vi "PSConverter.vi"(1 "Current States 2":string[][](table), 2 "PROC":string[](array[string]), 3 "STATES":string[][](array[string]), 4 "Input claster":cluster{u32, u8}[](array[cluster])) -> (0 "Current States":string[][](table))   [LabVIEW 2009]
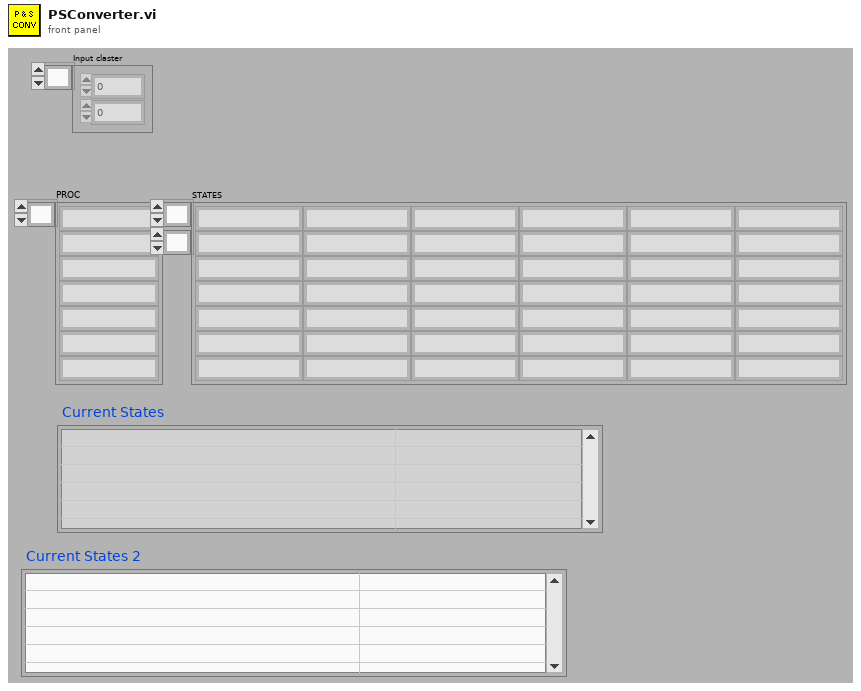
[diagram p1: front panel]
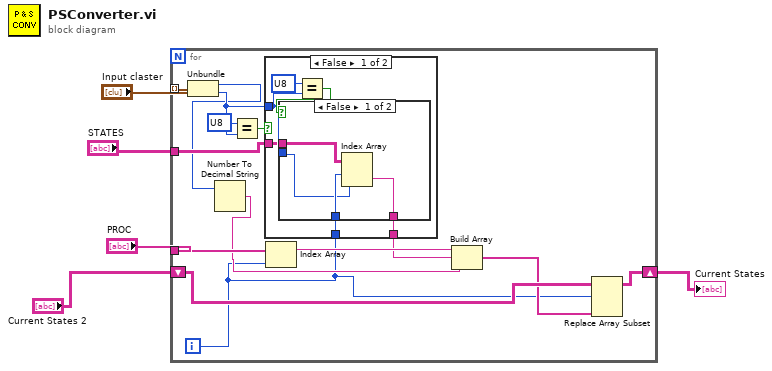
[diagram p0: block diagram]
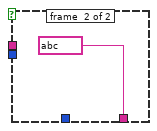
[diagram p2: hidden frame]
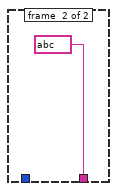
[diagram p3: hidden frame]
diagram:
  n1 = for {
    tunnel: "Input claster" -> [w19] mode=indexing
    tunnel: "PROC" -> [w13]
    tunnel: "STATES" -> [w12]
    shift-right: [w8] -> w5
    shift-left: "Current States 2" -> [w9]
    i -> [w6]
    n2 = Unbundle(w19) -> (w11:u32, w15:u8)
    n3 = Number To Decimal String(number=w11) -> (decimal integer string=w10:string)  [unwired: 1 in]
    n4 = Equal?(x=u8 ?, y=w15) -> (x = y?=w16:bool)
    n5 = case shown="False" w16 {
      tunnel: w15 -> [w21 _]
      tunnel: [w23 string ?] -> w14
      tunnel: w6 -> [w22 _]
      tunnel: w12 -> [w20 _]
      frame #0 {
        n6 = Equal?(x=u8 ?, y=w21) -> (x = y?=w24:bool)
        n7 = case shown="False" w24 {
          tunnel: [w27 string ?] -> w23
          tunnel: w22 -> [w29 _]
          tunnel: w21 -> [w28 _]
          tunnel: w20 -> [w26 _]
          frame #0 {
            n8 = Index Array(array=w26, index (row)=w29, index (col)=w28) -> (element=w27:string)
          }
          frame #1 {
          }
        }
      }
      frame #1 {
      }
    }
    n9 = Index Array(array=w13, index=w6) -> (element=w18:string)
    n10 = Build Array(w18, w14, w10) -> (w7:string[])
    n11 = Replace Array Subset(array=w9, new element=w7, index (row)=w6) -> (w8:string[][])  [unwired: 1 in]
  }
  "Current States" <- w5
